vi "Conn getDataToModify.vi"(4 "error in (no error)":errorcluster, 5 "ms timeout (-1)":i32=-1, 7 "connection reference":T2) -> (0 "error out":errorcluster, 1 "timed out":bool, 2 "data":T1, 3 "connection reference out":T2)   [LabVIEW 2017, in "NI_Database_API.lvlib"]
doc: "This VI returns the data associated with the <B>Connection</B> object reference and places a lock on the object.\n\nIf the object is currently locked for modification by another method, <B>timeout</B> specifies how long the VI should wait to receive access to the object. The default value waits until the object becomes available.\n\nIf the object does not become available for modification during <B>timeout</B> milliseconds, <B>timed out</B> will return TRUE.\n\nIf, and only if, you successfully locked the object's data for modification (i.e. <B>timed out</B> returned FALSE), you must use the <B>Connection Set Modified Data</B> VI to set the object's data and release the lock.\n\n[GOOP 1.0/1.0]"
uses:
  <vilib>/addons/database/NI_Database_API.lvlib
  <vilib>/addons/database/Connection.llb/Conn DataMembers.ctl
  <vilib>/addons/database/Connection.llb/Conn ObjectReference.ctl
  <vilib>/Utility/_goopsup.llb/GOOP Object Repository Method.ctl
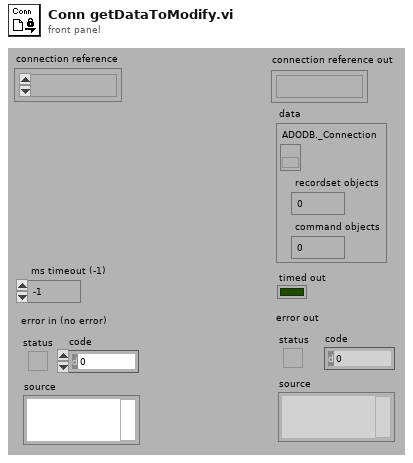
[diagram p1: front panel]
types:
  T1 = typedef "NI_Database_API.lvlib/Conn DataMembers.ctl" = cluster{"ADODB._Connection":refnum<k7>, "recordset objects":i32, "command objects":i32}
  T2 = typedef "NI_Database_API.lvlib/Conn ObjectReference.ctl" = refnum<k1>
  T3 = typedef "GOOP Object Repository Method.ctl" = enum16{"Create", "GetCopy", "GetModify", "Set", "Destroy", "Create Static", "Get All Refs", "Reset", "Get Statistics"}
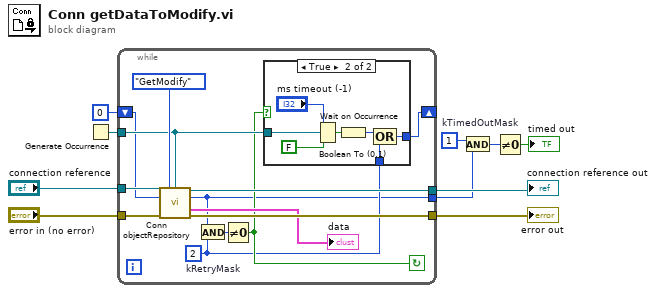
[diagram p0: block diagram]
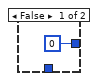
[diagram p2: hidden frame]
diagram:
  w4 = 1  # kTimedOutMask
  n1 = Generate Occurrence() -> (w6:refnum<k4>)
  n2 = while {
    tunnel: "error in (no error)" -> [w11]
    tunnel: [w12] -> w3
    tunnel: w6 -> [w18]
    shift-left: 0 -> [w16]
    shift-right: [w13] -> _
    tunnel: [w22] -> w2
    tunnel: [w23] -> w9
    tunnel: "connection reference" -> [w21]
    stop <- w15 continue-if-true
    w14 = 2  # kRetryMask
    n3 = call <vilib>:"Conn objectRepository.vi"("connection reference"=w21, "method"=GOOP_Object_Repository_Method."GetModify", "occurrence"=w18, "flags in"=w16, "error in (no error)"=w11) -> ("connection reference out"=w23:T2, "flags out"=w12:i32, "classDataOut"=→"data":T1, "error out"=w22:errorcluster)  [unwired: 4 in, 3 out]
    n4 = And(x=w12, y=w14) -> (x .and. y?=w17:i32)
    n5 = Not Equal To 0?(x=w17) -> (x != 0?=w15:bool)
    n6 = case shown="True" w15 {
      tunnel: w18 -> [_ w29]
      tunnel: w14 -> [_ w26]
      tunnel: [0 w25] -> w13
      frame False {
      }
      frame True {
        n7 = Wait on Occurrence(1:FALSE ("ignore previous (T)"), 2:w29, 3:"ms timeout (-1)") -> (0:w27:bool)
        n8 = Boolean To (0,1)(Boolean=w27) -> (0, 1=w28:i16)
        n9 = Compound Arithmetic op=OR(w28, w26) -> (w25:i32)
      }
    }
  }
  "error out" <- w2
  "connection reference out" <- w9
  n10 = And(x=w4, y=w3) -> (x .and. y?=w5:i32)
  n11 = Not Equal To 0?(x=w5) -> (x != 0?=→"timed out":bool)
